vi "Day 6.1 - .vi"(11 "input":string) -> (3 "output":i16)   [LabVIEW 2021]
panel:
  # "bvwbjplbgvbhsrlpgdmjqwftvncz: first marker after character 5\nnppdvjthqldpwncqszvftbrmjlhg: first marker after character 6\nnznrnfrfntjfmvfwmzdfjlvtqnbhcprsg: first marker after character 10\nzcfzfwzzqfrljwzlrfnpqdbhtmscgvjw: first marker after character 11"
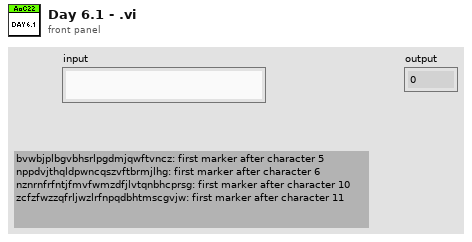
[diagram p1: front panel]
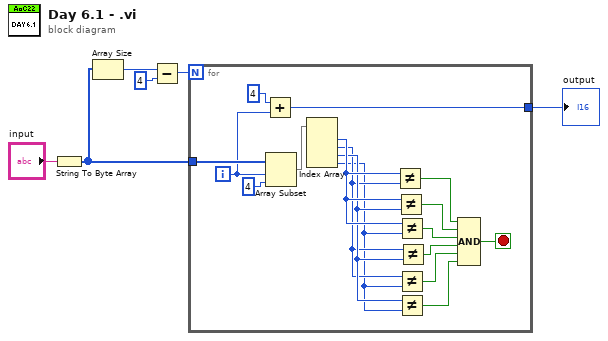
[diagram p0: block diagram]
diagram:
  n1 = String To Byte Array(string="input") -> (unsigned byte array=w1:u8[])
  n2 = Array Size(array=w1) -> (size(s)=w5:i32)
  n3 = Subtract(x=w5, y=4) -> (x-y=w3:i32)
  n4 = for {
    N: w3 -> [_]
    tunnel: w1 -> [w23]
    tunnel: [w20] -> w2
    i -> [w21]
    stop <- w7 stop-if-true
    n5 = Add(x=4, y=w21) -> (x+y=w20:i32)
    n6 = Array Subset(array=w23, index=w21, length=4) -> (w18:u8[])
    n7 = Index Array(array=w18) -> (element #1=w17:u8, element #2=w15:u8, element #3=w16:u8, element #4=w14:u8)  [unwired: 4 in]
    n8 = Not Equal?(x=w17, y=w15) -> (x != y?=w13:bool)
    n9 = Not Equal?(x=w17, y=w16) -> (x != y?=w12:bool)
    n10 = Not Equal?(x=w17, y=w14) -> (x != y?=w11:bool)
    n11 = Not Equal?(x=w15, y=w14) -> (x != y?=w9:bool)
    n12 = Not Equal?(x=w16, y=w14) -> (x != y?=w8:bool)
    n13 = Not Equal?(x=w15, y=w16) -> (x != y?=w10:bool)
    n14 = Compound Arithmetic op=AND(w13, w12, w11, w10, w9, w8) -> (w7:bool)
  }
  "output" <- w2
